vi "Set Server State Ref.vi"(10 "Server Internal State Ref":refnum<data-value>, 11 "Template Server in":refnum<class "Servicer.lvclass">) -> (3 "Template Server out":refnum<class "Servicer.lvclass">)   [LabVIEW 2019, in "gRPC-servicer.lvlib" / "Servicer.lvclass"]
uses:
  Servicer.lvclass
  typeDefs/Server State Data.ctl
  Servicer.lvclass/Servicer.ctl
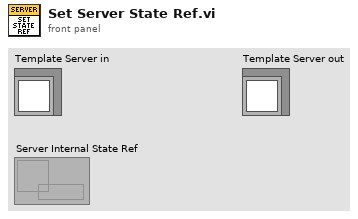
[diagram p1: front panel]
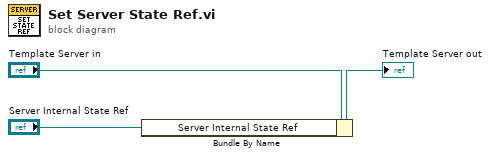
[diagram p0: block diagram]
diagram:
  n1 = Bundle By Name(cluster="Template Server in", "Server Internal State Ref"="Server Internal State Ref") -> (→"Template Server out":refnum<class "Servicer.lvclass">)
